vi "junk02.vi"() -> ()   [LabVIEW 2013]
uses:
  junkClass01.lvclass
panel:
  in  "stop":bool
  in  "Get Color":bool
  out "Color of Vehicle":u32(colorbox)
  in  "error in (no error)":errorcluster
  in  "Set Color":bool
  in  "Set Color":u32(colorbox)
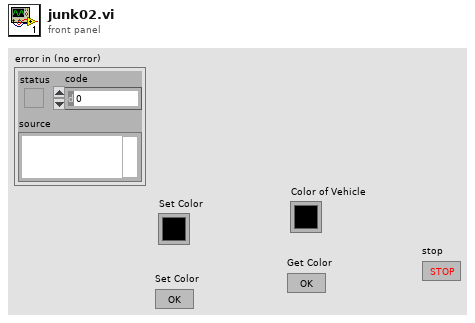
[diagram p1: front panel]
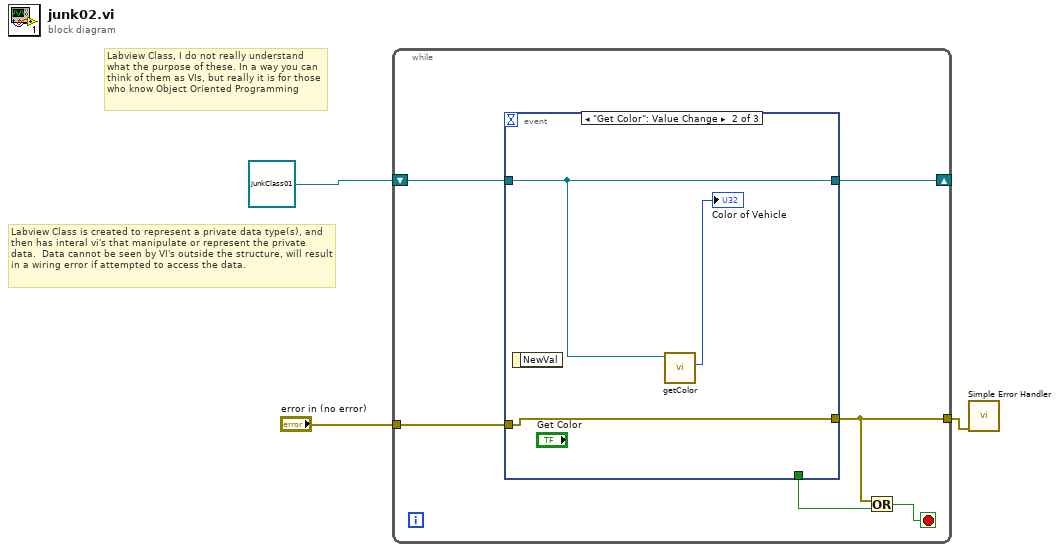
[diagram p0: block diagram]
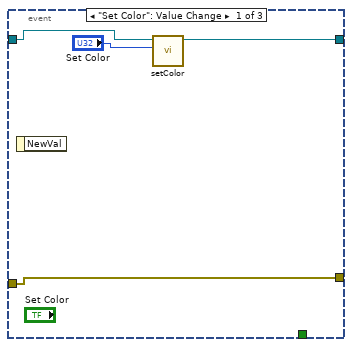
[diagram p2: hidden frame]
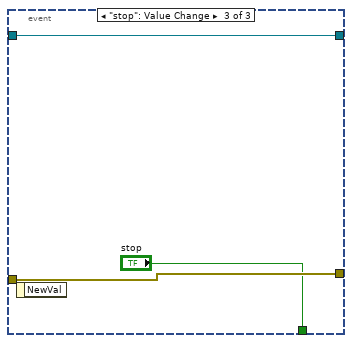
[diagram p3: hidden frame]
diagram:
  # "Labview Class is created to represent a private data type(s), and then has interal vi's that manipulate or represent the private data.  Data cannot be seen by VI's outside the structure, will result in a wiring error if attempted to access the data."
  # "Labview Class, I do not really understand what the purpose of these. In a way you can think of them as VIs, but really it is for those who know Object Oriented Programming"
  n1 = while {
    tunnel: "error in (no error)" -> [w9]
    tunnel: [w7] -> w2
    shift-right: [w5] -> _
    shift-left: refnum<class "junkClass01.lvclass"> refnum ("junkClass01.lvclass") -> [w4]
    stop <- w8 stop-if-true
    n2 = event shown="[1] \"Get Color\": Value Change" {
      selector: _ -> [_ _ _]
      dyn-events: _ -> [_ _ _]
      timeout: _ -> [_ _ _]
      tunnel: w9 -> [w13 w15 w19]
      tunnel: [w13 w15 w19] -> w7
      tunnel: [_ _ "stop"] -> w6
      tunnel: [w11 w14 w17] -> w5
      tunnel: w4 -> [w10 w14 w17]
      event "Set Color": Value Change {
        n3 = event-data() -> ()  [unwired: 1 in, 1 out]
        n4 = call-dynamic "setColor.vi"("Color Box"="Set Color", "junkClass01 in"=w10) -> ("junkClass01 out"=w11:refnum<class "junkClass01.lvclass">)  [unwired: 8 in, 1 out]
      }
      event "Get Color": Value Change {
        n5 = event-data() -> ()  [unwired: 1 in, 1 out]
        n6 = call-dynamic "getColor.vi"("junkClass01 in"=w14) -> ("Color Box"=→"Color of Vehicle":u32)  [unwired: 8 in, 2 out]
      }
      event "stop": Value Change {
        n7 = event-data() -> ()  [unwired: 1 in, 1 out]
      }
    }
    n8 = Or(x=w7, y=w6) -> (x .or. y?=w8:bool)
  }
  n9 = call <vilib>:"Simple Error Handler.vi"("error in (no error)"=w2) -> ()  [unwired: 4 in, 5 out]
